vi "Fetch LLB Documentation.vi"(5 "Parser Settings":T1, 8 "error in (no error)":errorcluster {"code" format="Error %.0f"}, 9 "Name":string, 11 "VI References":refnum<vi>[](array[refnum])) -> (0 "error out":errorcluster {"code" format="Error %.0f"}, 3 "LLB Documentation Out":refnum<class "LLB Documentation.lvclass">)   [LabVIEW 2023, in "VIDoc Parsing.lvlib" / "LLB Documentation.lvclass"]
doc: "Takes a VI Reference in and parses out all VI/UI Documentation information needed for document generation."
uses:
  LLB Documentation.lvclass
  Settings/Parser Settings/Parser Settings Cluster.ctl
  Settings/Parser Settings/Draw Controls Cluster.ctl
  Settings/Parser Settings/Draw Option Enum.ctl
  LLB Documentation.lvclass/LLB Documentation.ctl
  VIDoc Parsing.lvlib
  Settings/Parser Settings/Parser Settings.lvclass
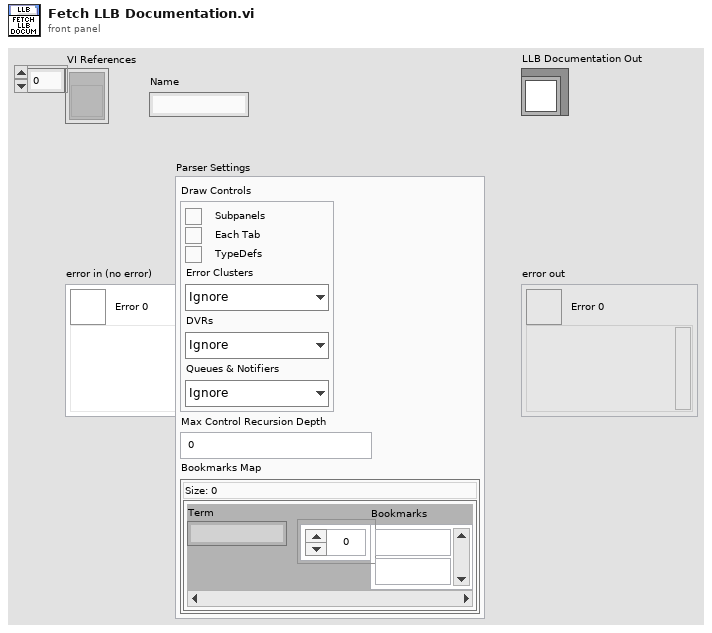
[diagram p1: front panel]
types:
  T1 = typedef "VIDoc Parsing.lvlib/Parser Settings.lvclass/Parser Settings Cluster.ctl" = cluster{"Draw Controls":T2, "Max Control Recursion Depth":i32, "Bookmarks Map":map{string, string[]}}
  T2 = typedef "VIDoc Parsing.lvlib/Parser Settings.lvclass/Draw Controls Cluster.ctl" = cluster{"Subpanels":bool, "Tabs":bool, "TypeDefs":bool, "Error Clusters":T3, "DVRs":T3, "Queues & Notifiers":T3}
  T3 = typedef "VIDoc Parsing.lvlib/Parser Settings.lvclass/Draw Option Enum.ctl" = enum16{"Ignore", "Draw", "Draw + Contents"}
  T4 = typedef "VIDoc Parsing.lvlib/Method Spec Cluster.ctl" = cluster{"VI Type Ext":T5, "Name":string, "Path":path, "Get Conpane Image":T6, "Description":string, "Get Library Access Scope":enum32{"invalid scope", "public", "private", "protected", "community"}, "Dispatch":T7, "ContainsCompiledCode":bool, "Exec.IsReentrant":bool, "Exec.ReentrancyType":enum16{"Share clones between instances", "Preallocate clone for each instance"}, "ExecInlining":bool, "ExecInlineIfPossible":bool, "Auto Err Handling":bool, "CodeComplexity":sgl, "Bookmark Tags":string[], "Control VI Type":enum32{"not a control VI", "control", "typedef", "strict typedef"}, "Controls":T8[], "VI Type":enum32{"invalid VI type", "Standard VI", "Control VI", "Global VI", "Polymorphic VI", "Configuration VI", "SubSystem", "Facade VI", "Method VI", "Statechart Diagram VI"}, "Minimum Size":T10, "Front Panel Window:Title":string, "Front Panel Window:Behavior":enum32{"Invalid", "Default", "Floating", "Floating/Auto-Hide", "Modal"}, "Front Panel Window:Closeable":bool, "Must Override":bool, "Must Use Parent Implementation":bool, "VI Icon":T6, "Front Panel":T6, "History:Revision Number":u32, "Metrics:Total Data Size":u32, "Execution:Allow Debugging":bool, "Execution:Preferred Exec System":enum32{"invalid execution system", "user interface", "standard", "instrument i/o", "data acquisition", "other 1", "other 2", "same as caller"}, "Execution:Priority":enum32{"invalid priority", "background priority", "normal priority", "above normal priority", "high priority", "time critical priority", "subroutine"}, "BM Tag Text":string[], "Block Diagram":T6, "Structure Tree":T11[]}
  T5 = typedef "VIDoc Parsing.lvlib/VI Type Extended Enum.ctl" = enum16{"Unknown", "Class Method", "Class Accessor Get", "Class Accessor Set", "Class Control", "Library Method", "Library Control", "VI", "Control"}
  T6 = typedef "imagedata.ctl" = cluster{"image type":i32, "image depth":i32, "image":u8[], "mask":u8[], "colors":u32[], "Rectangle":cluster{"left":i16, "top":i16, "right":i16, "bottom":i16}}
  T7 = typedef "VIDoc Parsing.lvlib/Class Dispatch Type Enum.ctl" = enum16{"None", "Static", "Dynamic"}
  T8 = typedef "VIDoc Parsing.lvlib/Controls Info Cluster.ctl" = cluster{"Name":string, "Description":string, "Data Type":string, "Tip Strip":string, "UID":i32, "Image Data":T6, "ToggleKeyBind":T9, "Raw Label":string, "Raw Caption":string}
  T9 = typedef "LVKeyTypeDef.ctl" = cluster{"Focus":bool, "Control":bool, "Shift":bool, "Key":string}
  T10 = typedef "LVPointTypeDef.ctl" = cluster{"Horizontal":i16, "Vertical":i16}
  T11 = typedef "VIDoc Parsing.lvlib/Structure Reporter.lvlib/Tree Cluster.ctl" = cluster{"Object Class Name":string, "Labels":string[], "Child Tag":string, "Item Indent":i32, "Child Only?":bool, "Glyph Index":i32}
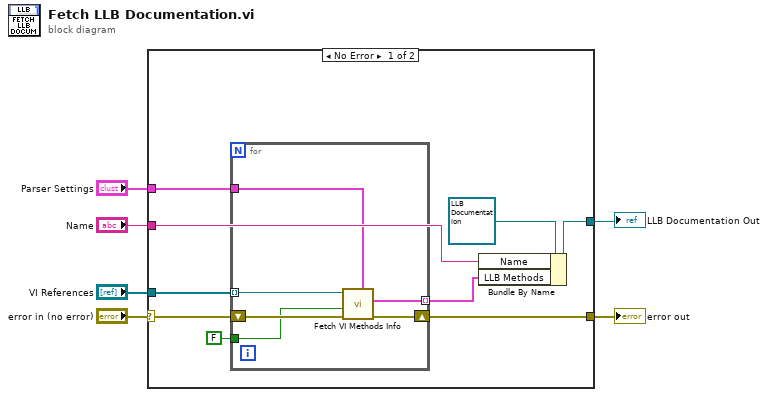
[diagram p0: block diagram]
diagram:
  n1 = case shown="No Error" "error in (no error)" {
    selector: "error in (no error)" -> [w13 w22]
    tunnel: [w12 w22] -> w5
    tunnel: [w15 _] -> w4
    tunnel: "VI References" -> [w14 _]
    tunnel: "Parser Settings" -> [w11 _]
    tunnel: "Name" -> [w8 _]
    frame No Error {
      n2 = for {
        tunnel: w14 -> [w21] mode=indexing
        tunnel: w11 -> [w18]
        tunnel: FALSE ("Fetch Controls?") -> [w17]
        shift-right: [w19] -> w12
        shift-left: w13 -> [w20]
        tunnel: [w16] -> w9 mode=indexing
        n3 = call "Fetch VI Methods Info.vi"("Parser Settings"=w18, "Error in"=w20, "Fetch Controls?"=w17, "VI Reference"=w21) -> ("Error out"=w19:errorcluster, "VI Info"=w16:T4)  [unwired: 6 in]
      }
      n4 = Bundle By Name(cluster=refnum<class "LLB Documentation.lvclass"> refnum ("Documentation Parsing.lvlib:LLB Documentation.lvclass"), "Name"=w8, "LLB Methods"=w9) -> (w15:refnum<class "LLB Documentation.lvclass">)
    }
    frame Error {
    }
  }
  "error out" <- w5
  "LLB Documentation Out" <- w4
